vi "Requirements_application.vi"(6 "Static values":T5, 8 "error_in":errorcluster, 10 "Data Model":T2={"Time_control"=[], "P_ch_av (from grid)"=[], "PV_exc (W)"=[], "PV_exc (Wh)"=[], "Delta_t"=0.0, "Timestamp"=0, "SOC_end (array)"=[], "SOC_ini (array)"=[], "SOC_max_min"=[], "N_periods"=0, "SOC_end"=[], "SOC_ini"=[], "t_end"=[], "t_ini"=[], "Plugged"=[], "P_charge vs. SOC"={"SOC"=[0.0, 100.0], "P"=[3700.0, 3700.0]}, "SOC_ini_save"=[], "SOC_ini_save (array)"=[]}, 11 "Requirements":T4) -> (0 "error_out":errorcluster, 1 "SOC_reqs":T1, 2 "Data Model":T2={"Time_control"=[], "P_ch_av (from grid)"=[], "PV_exc (W)"=[], "PV_exc (Wh)"=[], "Delta_t"=0.0, "Timestamp"=0, "SOC_end (array)"=[], "SOC_ini (array)"=[], "SOC_max_min"=[], "N_periods"=0, "SOC_end"=[], "SOC_ini"=[], "t_end"=[], "t_ini"=[], "Plugged"=[], "P_charge vs. SOC"={"SOC"=[0.0, 100.0], "P"=[3700.0, 3700.0]}, "SOC_ini_save"=[], "SOC_ini_save (array)"=[]})   [LabVIEW 2017]
uses:
  CONTROLS/Static_values.ctl
  CONTROLS/Requirements.ctl
  CONTROLS/Datamodel_FULL.ctl
  CONTROLS/P_ch_vs_SOC (array).ctl
  CONTROLS/SOC_reqs.ctl
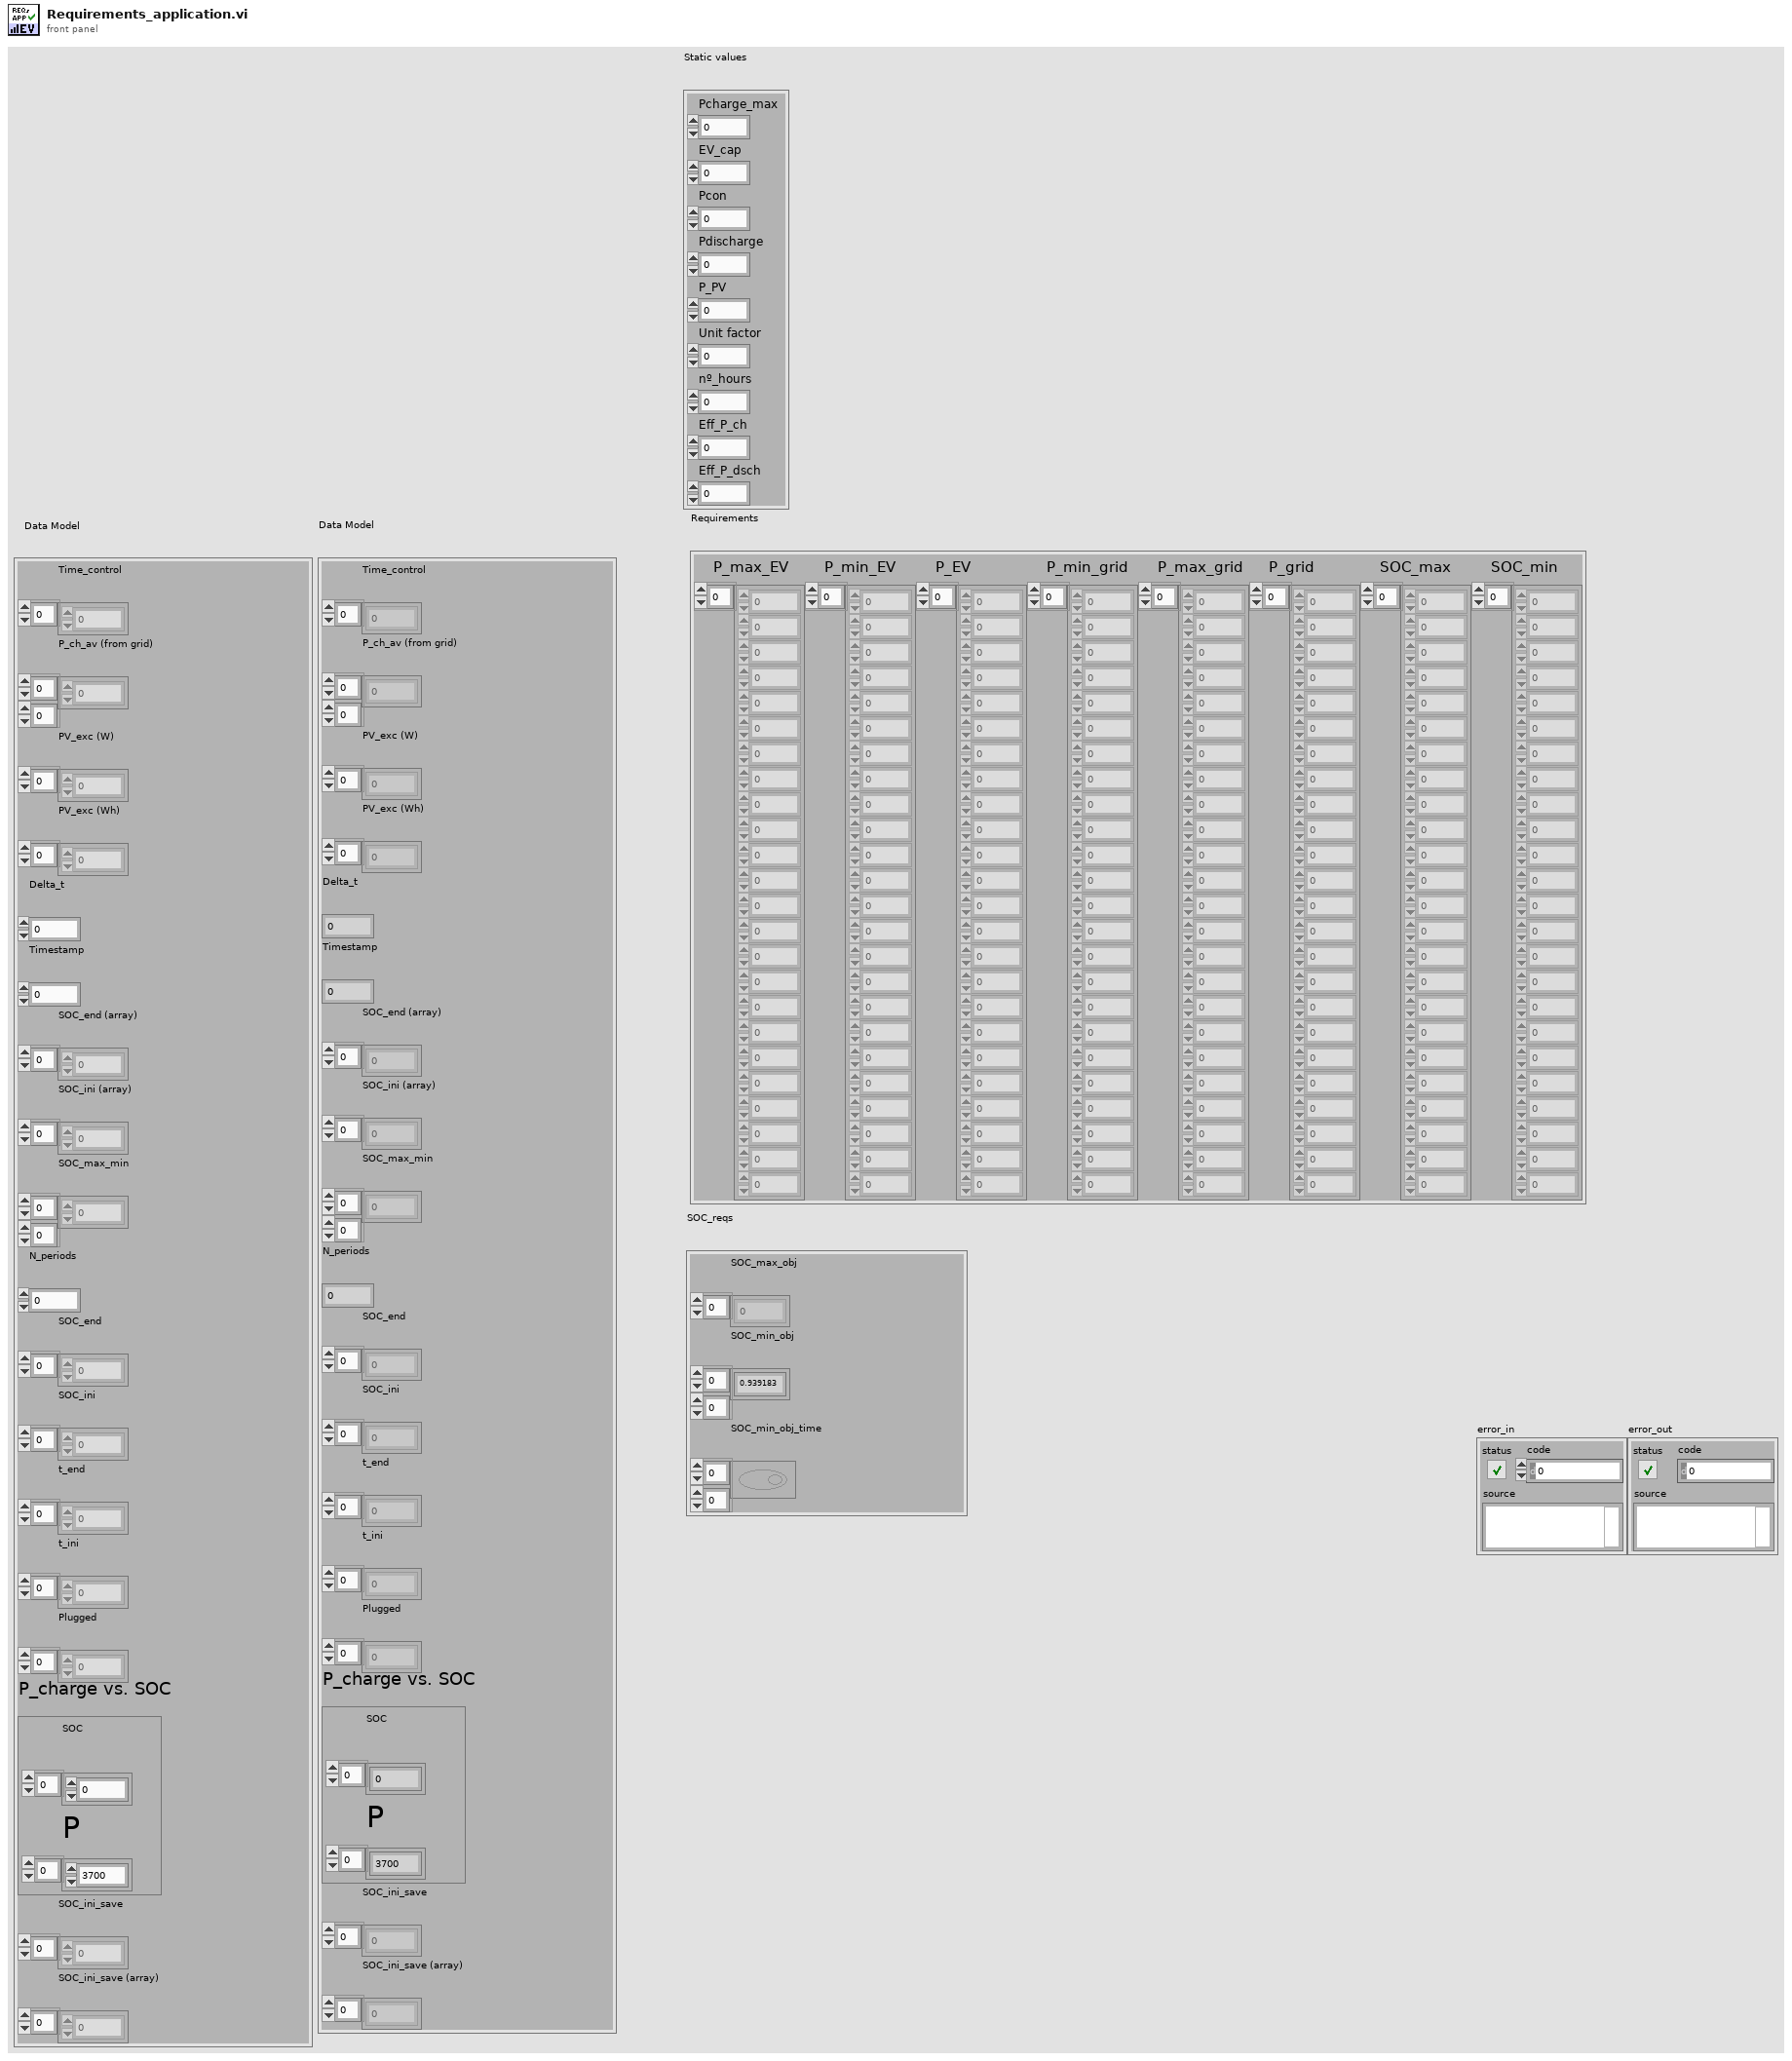
[diagram p1: front panel]
types:
  T1 = typedef "SOC_reqs.ctl" = cluster{"SOC_max_obj":dbl[], "SOC_min_obj":dbl[][], "SOC_min_obj_time":bool[][]}
  T2 = typedef "Datamodel_FULL.ctl" = cluster{"Time_control":i32[], "P_ch_av (from grid)":dbl[][], "PV_exc (W)":dbl[], "PV_exc (Wh)":dbl[], "Delta_t":dbl, "Timestamp":i32, "SOC_end (array)":dbl[], "SOC_ini (array)":dbl[], "SOC_max_min":dbl[][], "N_periods":i32, "SOC_end":dbl[], "SOC_ini":dbl[], "t_end":i32[], "t_ini":i32[], "Plugged":i32[], "P_charge vs. SOC":T3, "SOC_ini_save":dbl[], "SOC_ini_save (array)":dbl[]}
  T3 = typedef "P_ch_vs_SOC (array).ctl" = cluster{"SOC":dbl[], "P":dbl[]}
  T4 = typedef "Requirements.ctl" = cluster{"P_max_EV":dbl[], "P_min_EV":dbl[], "P_EV":dbl[], "P_min_grid":dbl[], "P_max_grid":dbl[], "P_grid":dbl[], "SOC_max":dbl[], "SOC_min":dbl[]}
  T5 = typedef "Static_values.ctl" = cluster{"Pcharge_max":dbl, "EV_cap":dbl, "Pcon":dbl, "Pdischarge":dbl, "P_PV":dbl, "Unit factor":dbl, "nº_hours":dbl, "Eff_P_ch":dbl, "Eff_P_dsch":dbl}
  T6 = typedef "Requirements_boolean.ctl" = cluster{"P_max_EV":bool[], "P_min_EV":bool[], "P_EV":bool[], "P_min_grid":bool[], "P_max_grid":bool[], "P_grid":bool[], "SOC_max":bool[], "SOC_min":bool[], "Any?":bool}
  T7 = typedef "Reqs_cluster.ctl" = cluster{"E_max":dbl[], "E_min":dbl[], "P_max_EV":dbl[], "P_min_EV":dbl[], "P_max_grid":dbl[], "P_min_grid":dbl[]}
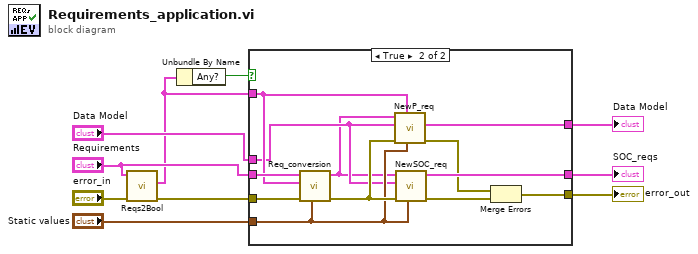
[diagram p0: block diagram]
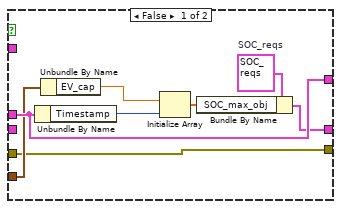
[diagram p2: hidden frame]
diagram:
  n1 = call "Reqs2Bool.vi"("error_in"="error_in", "Requirements"="Requirements") -> ("error_out"=w2:errorcluster, "Requeriments_boolean"=w4:T6)  [unwired: 8 in]
  n2 = Unbundle By Name(w4) -> ("Any?"=w5:bool)
  n3 = case shown="True" w5 {
    tunnel: "Data Model" -> [w18 w21]
    tunnel: [w18 w20] -> w9
    tunnel: "Static values" -> [w17 w22]
    tunnel: [w14 w23] -> w7
    tunnel: w2 -> [w14 w29]
    tunnel: "Requirements" -> [_ w30]
    tunnel: w4 -> [_ w28]
    tunnel: [w11 w27] -> w1
    frame False {
      w13 = T1 {"SOC_max_obj"=[], "SOC_min_obj"=array1x86400[86400 elements], "SOC_min_obj_time"=[]}  # SOC_reqs
      n4 = Unbundle By Name(w18) -> ("Timestamp"=w15:i32)
      n5 = Unbundle By Name(w17) -> ("EV_cap"=w16:dbl)
      n6 = Initialize Array(w16, w15) -> (w12:dbl[])
      n7 = Bundle By Name(cluster=w13, "SOC_max_obj"=w12) -> (w11:T1)
    }
    frame True {
      n8 = call "Req_conversion.vi"("Static values in"=w22, "error_in"=w29, "reqs_bool"=w28, "Requirements"=w30) -> ("error_out"=w26:errorcluster, "Reqs_cluster"=w19:T7)  [unwired: 5 in]
      n9 = call "NewP_req.vi"("Static values"=w22, "Requeriments_boolean"=w28, "error in (no error)"=w26, "Data Model in"=w21, "Reqs_cluster"=w19) -> ("error out"=w25:errorcluster, "Data Model out"=w20:T2)  [unwired: 5 in]
      n10 = call "NewSOC_req.vi"("Static values"=w22, "error_in"=w26, "Data Model"=w21, "Reqs_cluster"=w19) -> ("error_out"=w24:errorcluster, "SOC_reqs"=w27:T1)  [unwired: 6 in]
      n11 = Merge Errors(w25, w24) -> (w23:errorcluster)
    }
  }
  "error_out" <- w7
  "Data Model" <- w9
  "SOC_reqs" <- w1
